vi "list.free.vi"(8 "error in":errorcluster, 11 "List in":refnum<class "List.lvclass">) -> (0 "error out":errorcluster)   [LabVIEW 2020, in "List.lvclass"]
uses:
  List.lvclass
  List.lvclass/List.ctl
  client.lvlib
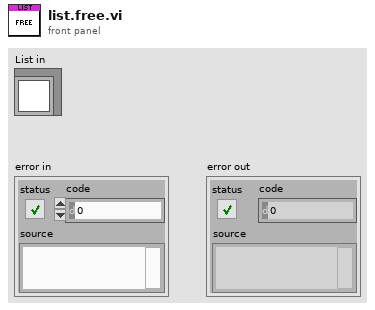
[diagram p1: front panel]
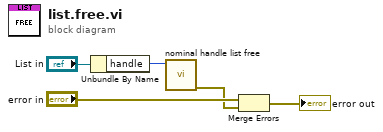
[diagram p0: block diagram]
diagram:
  n1 = Unbundle By Name("List in") -> ("handle"=w3:i32)
  n2 = call "nominal handle list free.vi"("list"=w3) -> ("error out"=w2:errorcluster)  [unwired: 9 in, 1 out]
  n3 = Merge Errors("error in", w2) -> (→"error out":errorcluster)
